vi "时间计算.vi"(8 "错误常量in":errorcluster caption="错误常量", 10 "运行状态":string, 11 "实时压力":string) -> (0 "错误常量out":errorcluster caption="错误常量")   [LabVIEW 2015]
uses:
  <userlib>/_OpenG.lib/comparison/comparison.llb/String Changed__ogtk.vi
  Global.vi
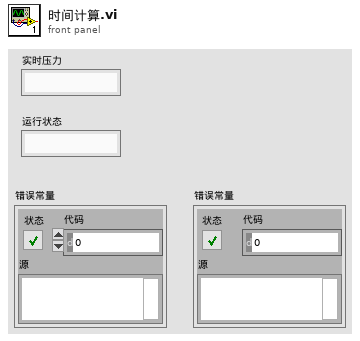
[diagram p1: front panel]
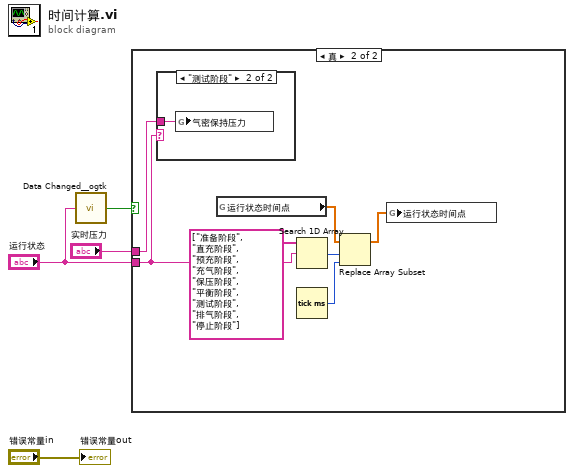
[diagram p0: block diagram]
diagram:
  n1 = call-poly <userlib>:"Data Changed__ogtk.vi"("String"="运行状态") -> ("Changed"=w4:bool)
  n2 = case shown="真" w4 {
    tunnel: "运行状态" -> [_ w10]
    tunnel: "实时压力" -> [_ w11]
    frame False {
    }
    frame True {
      n3 = case shown="\"测试阶段\"" w10 {
        tunnel: w11 -> [_ w12]
        frame "假", Default {
        }
        frame "测试阶段" {
          n4 = global write "Global.vi" "气密保持压力"(w12) -> ()
        }
      }
      n5 = global read "Global.vi" "运行状态时间点"() -> (w9:dbl[])
      n6 = Search 1D Array(1D array=string[] ["准备阶段", "直充阶段", "预充阶段", "充气阶段", "保压阶段", "平衡阶段", "测试阶段", "排气阶段", "停止阶段"], element=w10) -> (index of element=w5:i32)  [unwired: 1 in]
      n7 = Tick Count (ms)() -> (millisecond timer value=w8:u32)
      n8 = Replace Array Subset(array=w9, new element=w8, index=w5) -> (w6:dbl[])
      n9 = global write "Global.vi" "运行状态时间点"(w6) -> ()
    }
  }
  "错误常量out" <- "错误常量in"
